vi "create_project_vipc.vi"(6 "quet":bool=TRUE, 8 "error in (no error)":errorcluster, 10 "dependencies_folder":path, 11 "project_file":path) -> (0 "error out":errorcluster)   [LabVIEW 2015, in "lv-builder-default.lvlib"]
uses:
  lv-builder-default.lvlib
  <vilib>/JKI/VIPM API/VIPM API_vipm_api.lvlib
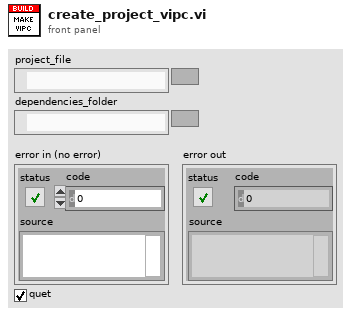
[diagram p1: front panel]
types:
  T1 = typedef "VIPM API_vipm_api.lvlib/LabVIEW Target Info Cluster_vipm_api.ctl" = cluster{"Version":string, "Connection Tested":bool, "Disabled":bool}
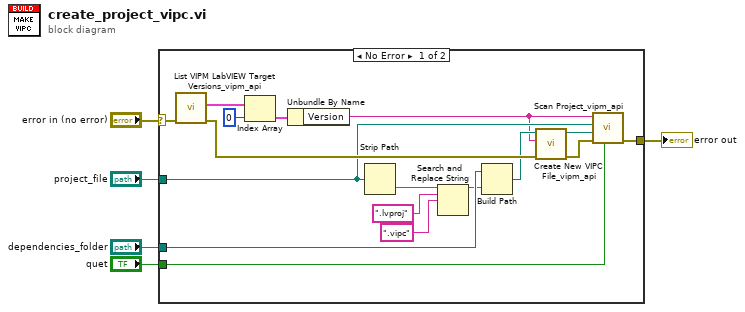
[diagram p0: block diagram]
diagram:
  n1 = case shown="No Error" "error in (no error)" {
    selector: "error in (no error)" -> [w10 w22]
    tunnel: "project_file" -> [w15 _]
    tunnel: [w20 w22] -> w3
    tunnel: "quet" -> [w19 _]
    tunnel: "dependencies_folder" -> [w16 _]
    frame No Error {
      n2 = call <vilib>:"List VIPM LabVIEW Target Versions_vipm_api.vi"("error in (no error)"=w10) -> ("error out"=w21:errorcluster, "LabVIEW Target Info"=w9:T1[])  [unwired: 9 in]
      n3 = Index Array(array=w9, index=0) -> (element=w8:T1)
      n4 = Unbundle By Name(w8) -> ("Version"=w7:string)
      n5 = Strip Path(path=w15) -> (name=w14:string)  [unwired: 1 out]
      n6 = Search and Replace String(input string=w14, search string=".lvproj" ("regular expression"), replace string=".vipc" ("string")) -> (result string=w13:string)  [unwired: 5 in, 3 out]
      n7 = Build Path(base path=w16, name or relative path=w13) -> (appended path=w17:path)
      n8 = call <vilib>:"Create New VIPC File_vipm_api.vi"("error in (no error)"=w21, "LabVIEW Version"=w7, "Path to New VIPC File"=w17) -> ("error out"=w18:errorcluster)  [unwired: 8 in]
      n9 = call <vilib>:"Scan Project_vipm_api.vi"("quiet? (T)"=w19, "error in (no error)"=w18, "Path to VIPC File"=w17, "Project file, VI or project dir path"=w15, "LabVIEW Version"=w7) -> ("error out"=w20:errorcluster)  [unwired: 6 in]
    }
    frame Error {
    }
  }
  "error out" <- w3
